vi "Modes and States 2017.vi"(11 "All Robot Commands In":T5) -> (3 "All Robot Commands Out":T5)   [LabVIEW 2016]
uses:
  Drive and Climb SS/Drive + Climb Commands 2017.ctl
  Gear Delivery SS/Gear Delivery Commands.ctl
  Conveyor and Shooter SS/Conveyor and Shooter Commands.ctl
  Ball Intake SS/Ball Intake Commands.ctl
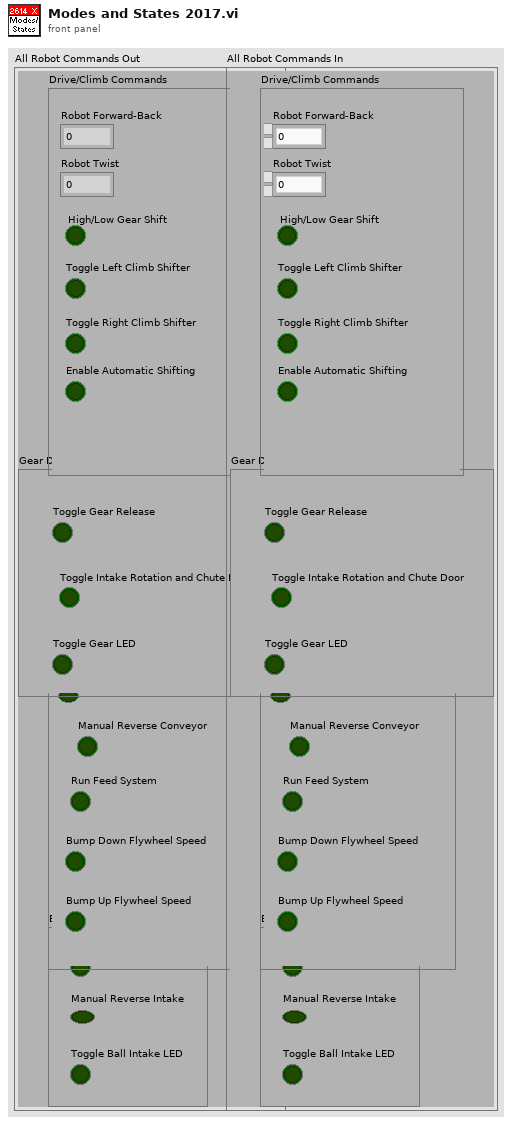
[diagram p1: front panel]
types:
  T1 = typedef "Drive + Climb Commands 2017.ctl" = cluster{"Robot Forward-Back":dbl, "Robot Twist":dbl, "High/Low Gear Shift":bool, "Toggle Left Climb Shifter":bool, "Toggle Right Climb Shifter":bool, "Enable Automatic Shifting":bool}
  T2 = typedef "Gear Delivery Commands.ctl" = cluster{"Toggle Gear Release":bool, "Toggle Intake Rotation and Chute Door":bool, "Toggle Gear LED":bool}
  T3 = typedef "Conveyor and Shooter Commands.ctl" = cluster{"Toggle Shooter":bool, "Manual Reverse Conveyor":bool, "Run Feed System":bool, "Bump Down Flywheel Speed":bool, "Bump Up Flywheel Speed":bool}
  T4 = typedef "Ball Intake Commands.ctl" = cluster{"Toggle Ball Intake":bool, "Manual Reverse Intake":bool, "Toggle Ball Intake LED":bool}
  T5 = cluster{"Drive/Climb Commands":T1, "Gear Delivery Commands":T2, "Shooter and Conveyor Commands":T3, "Ball Intake Commands":T4}
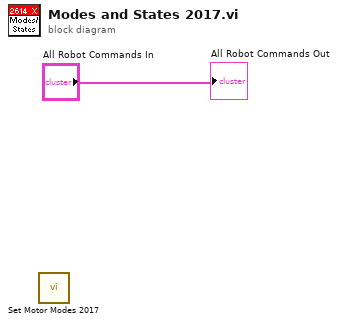
[diagram p0: block diagram]
diagram:
  n1 = call "Set Motor Modes 2017.vi"() -> ()  [unwired: 12 in]
  "All Robot Commands Out" <- "All Robot Commands In"
